vi "BH1750 Read.vi"(7 "I2C Channel (0)":u8, 8 "error in (no error)":errorcluster, 9 "Resoultion (lux)":dbl, 10 "BH1750address":u8, 11 "LINX Resource in":T1) -> (0 "error out":errorcluster, 1 "64 bit value":u16, 2 "Lux value":dbl, 3 "LINX Resource":T1)   [LabVIEW 2022 SP3]
uses:
  <vilib>/MakerHub/LINX/Private/Type Defs/LINX Ref.ctl
  <vilib>/MakerHub/LINX/Private/Type Defs/Platform.ctl
  <vilib>/MakerHub/LINX/Private/Type Defs/Interface.ctl
  <vilib>/MakerHub/LINX/Private/Device/Type Defs/LINX Device Config.ctl
  <vilib>/MakerHub/LINX/Private/Device/Type Defs/TCP Config.ctl
  <vilib>/MakerHub/LINX/Private/Device/Type Defs/Channels.ctl
  <vilib>/MakerHub/LINX/LMH-LINX.lvlib
  <vilib>/MakerHub/LINX/Private/Device/Device.lvlib
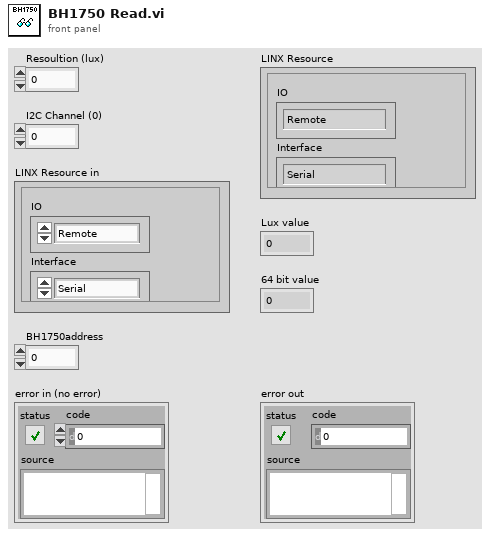
[diagram p1: front panel]
types:
  T1 = typedef "LMH-LINX.lvlib/LINX Ref.ctl" = cluster{"IO":T2, "Interface":T3, "LINX Device Config":T4}
  T2 = typedef "LMH-LINX.lvlib/Platform.ctl" = enum16{"Remote", "Local"}
  T3 = typedef "LMH-LINX.lvlib/Interface.ctl" = enum16{"Serial", "TCP"}
  T4 = typedef "LMH-LINX.lvlib/Device.lvlib/LINX Device Config.ctl" = cluster{"Interface":T3, "COM Port":refnum<visa-resource-name>, "TCP Configuration":T5, "Device Family":u8, "Device ID":u8, "Device Name":string, "TCP Ref":refnum<k5>, "Channels":T6}
  T5 = typedef "LMH-LINX.lvlib/Device.lvlib/TCP Config.ctl" = cluster{"IP Address":string, "Port":u16}
  T6 = typedef "LMH-LINX.lvlib/Channels.ctl" = cluster{"DI":u8[], "DO":u8[], "AI":u8[], "AO":u8[], "PWM":u8[], "QE":u8[], "UART":u8[], "I2C 2":u8[], "SPI":u8[], "CAN":u8[], "Servo":u8[], "AI Ref (V)":dbl, "AI Resolution (Bits)":u8, "AO Ref (V)":dbl, "AO Resolution (Bits)":u8}
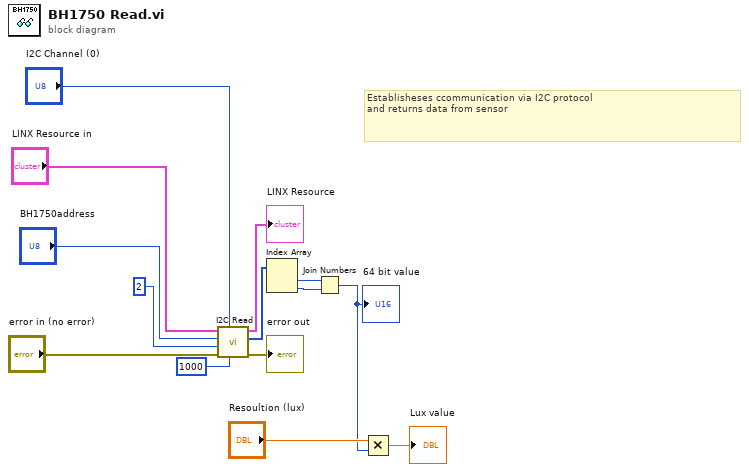
[diagram p0: block diagram]
diagram:
  # "Establisheses ccommunication via I2C protocol\nand returns data from sensor"
  n1 = call <vilib>:"I2C Read.vi"("Timeout (1000 ms)"=u16 1000, "I2C Channel"="I2C Channel (0)", "Error In"="error in (no error)", "Bytes To Read"=u8 2, "I2C Slave Address (0)"="BH1750address", "LINX Resource"="LINX Resource in") -> ("Error Out"=→"error out":errorcluster, "Data"=w9:u8[], "LINX Resource"=→"LINX Resource":T1)  [unwired: 3 in]
  n2 = Index Array(array=w9) -> (element #1=w11:u8, element #2=w10:u8)  [unwired: 2 in]
  n3 = Join Numbers(hi=w11, lo=w10) -> ((hi.lo)=w12:u16)
  "64 bit value" <- w12
  n4 = Multiply(x="Resoultion (lux)", y=w12) -> (x*y=→"Lux value":dbl)
